vi "example_main.vi"() -> ()   [LabVIEW 2015]
doc: "# #############################################################################\n# ATTENTION\n# #############################################################################\n#\n# This software is for guidance only. It is provided \"as is\".\n# It only aims at providing coding information to the customer in order for\n# them to save time. As a result no warranties, whether express, implied or\n# statutory, including, but not limited to implied warranties of\n# merchantability and fitness for a particular purpose apply to this software.\n# A·P·E Angewandte Physik und Elektronik GmbH shall not be held liable for any\n# direct, indirect or consequential damages with respect to any claims arising\n# from the content of such sourcecode and/or the use made by customers of the\n# coding information contained herein in connection with their products.\n#\n# File Version: 1.0\n#\n# Changelog:\n# 1.0 - Initial Version\n#\n# #############################################################################"
uses:
  <vilib>/Utility/miscctls.llb/LVPointTypeDef.ctl
  cluster/tcp client action.ctl
panel:
  in  "error in":errorcluster
  out "error out":errorcluster
  in  "Send":bool
  out "Answer":string
  in  "Command":string="*IDN?\n"
  in  "Connect":bool
  in  "Host":string="127.0.0.1"
  in  "Port":u16=51019
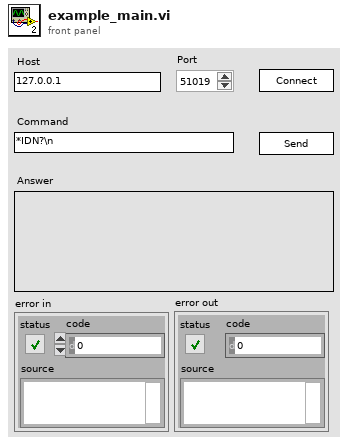
[diagram p1: front panel]
types:
  T1 = typedef "LVPointTypeDef.ctl" = cluster{"Horizontal":i16, "Vertical":i16}
  T2 = typedef "tcp client action.ctl" = enum16{"Connect", "Write", "Query", "Disconnect"}
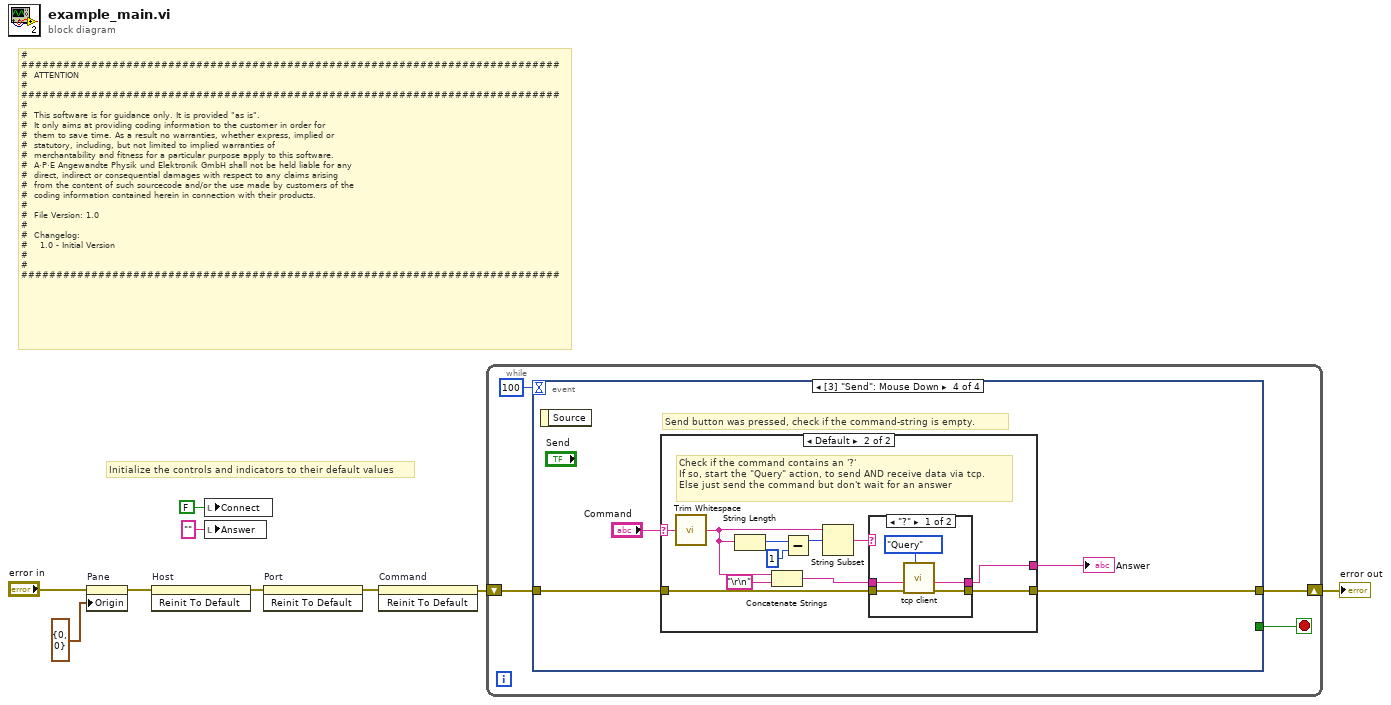
[diagram p0: block diagram]
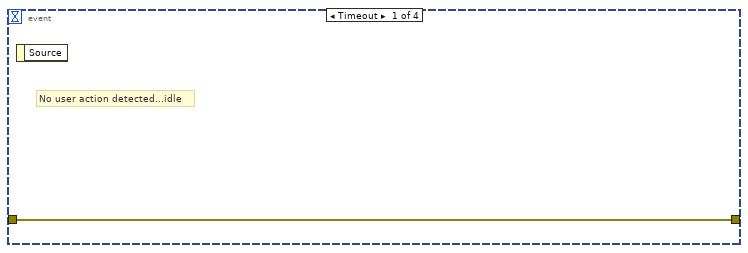
[diagram p2: hidden frame]
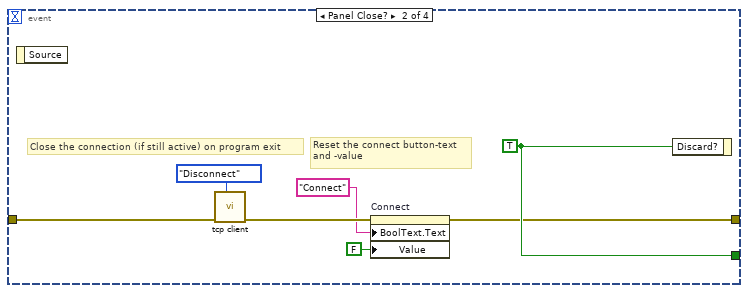
[diagram p3: hidden frame]
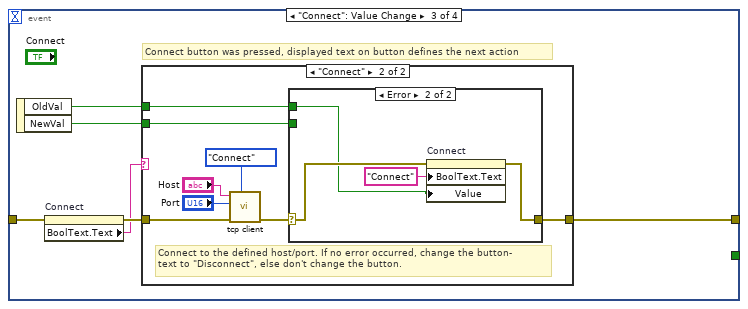
[diagram p4: hidden frame]
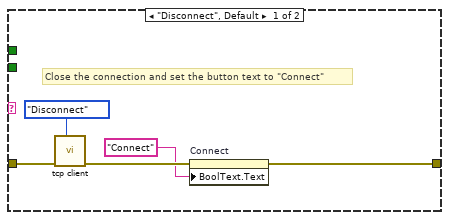
[diagram p5: hidden frame]
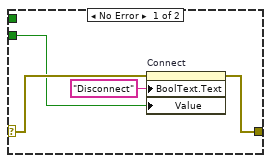
[diagram p6: hidden frame]
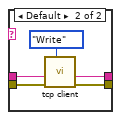
[diagram p8: hidden frame]
diagram:
  # "# #############################################################################\n#  ATTENTION\n# #############################################################################\n#\n#  This software is for guidance only. It is provided \"as is\".\n#  It only aims at providing coding information to the customer in order for\n#  them to save time. As a result no warranties, whether express, implied or\n#  statutory, including, but not limited to implied warranties of\n#  merchantability and fitness for a particular purpose apply to this software.\n#  A·P·E Angewandte Physik und Elektronik GmbH shall not be held liable for any\n#  direct, indirect or consequential damages with respect to any claims arising\n#  from the content of such sourcecode and/or the use made by customers of the\n#  coding information contained herein in connection with their products.\n#\n#  File Version: 1.0\n#\n#  Changelog:\n#    1.0 - Initial Version\n#\n# #############################################################################"
  # "Initialize the controls and indicators to their default values"
  n1 = property on="Pane" class="Pane"(error in="error in", "Origin"=T1 {"Horizontal"=0, "Vertical"=0}) -> (error out=w2:errorcluster)  [unwired: 1 in, 1 out]
  n2 = invoke on="Host" class="Str" method="Reinit To Default"(error in=w2) -> (error out=w5:errorcluster)  [unwired: 2 in, 2 out]
  n3 = local write "Connect"(FALSE ("Connect")) -> ()
  n4 = local write "Answer"("" ("Answer")) -> ()
  n5 = invoke on="Port" class="DigNum (strict)" method="Reinit To Default"(error in=w5) -> (error out=w4:errorcluster)  [unwired: 2 in, 2 out]
  n6 = invoke on="Command" class="Str" method="Reinit To Default"(error in=w4) -> (error out=w3:errorcluster)  [unwired: 2 in, 2 out]
  n7 = while {
    shift-right: [w12] -> w9
    shift-left: w3 -> [w11]
    stop <- w10 stop-if-true
    n8 = event shown="[3] \"Send\": Mouse Down" {
      selector: _ -> [_ _ _ _]
      dyn-events: _ -> [_ _ _ _]
      timeout: 100 -> [_ _ _ _]
      tunnel: w11 -> [w14 w21 w26 w52]
      tunnel: [w14 w17 w27 w49] -> w12
      tunnel: [_ w19 _ _] -> w10
      event Timeout {
        # "No user action detected...idle"
        n9 = event-data() -> ()  [unwired: 1 in, 1 out]
      }
      event Panel Close? {
        w19 = TRUE ("Discard?")
        # "Reset the connect button-text\nand -value"
        # "Close the connection (if still active) on program exit"
        n10 = event-data() -> ()  [unwired: 1 in, 1 out]
        n11 = call "tcp client.vi"("Action"=tcp_client_action."Disconnect", "error in"=w21) -> ("error out"=w18:errorcluster)  [unwired: 8 in, 1 out]
        n12 = property on="Connect" class="Bool (strict)"(error in=w18, "BoolText.Text"="Connect" ("Boolean Text.Text"), "Value"=FALSE ("Connect")) -> (error out=w17:errorcluster)  [unwired: 1 in, 1 out]
        n13 = event-data("Discard?"=w19) -> ()  [unwired: 1 in, 1 out]
      }
      event "Connect": Value Change {
        # "Connect button was pressed, displayed text on button defines the next action"
        n14 = event-data() -> ("OldVal"=w22:bool, "NewVal"=w23:bool)  [unwired: 1 in]
        n15 = property on="Connect" class="Bool (strict)"(error in=w26) -> (error out=w25:errorcluster, "BoolText.Text"=w24:string)  [unwired: 1 in, 1 out]
        n16 = case shown="\"Connect\"" w24 {
          tunnel: [w29 w36] -> w27
          tunnel: w25 -> [w31 w37]
          tunnel: w23 -> [_ w34]
          tunnel: w22 -> [_ w33]
          frame "Disconnect", Default {
            # "Close the connection and set the button text to \"Connect\""
            n17 = call "tcp client.vi"("Action"=tcp_client_action."Disconnect", "error in"=w31) -> ("error out"=w30:errorcluster)  [unwired: 8 in, 1 out]
            n18 = property on="Connect" class="Bool (strict)"(error in=w30, "BoolText.Text"="Connect" ("Boolean Text.Text")) -> (error out=w29:errorcluster)  [unwired: 1 in, 1 out]
          }
          frame "Connect" {
            # "Connect to the defined host/port. If no error occurred, change the button-\ntext to \"Disconnect\", else don't change the button."
            n19 = call "tcp client.vi"("Action"=tcp_client_action."Connect", "error in"=w37, "TCP Port"="Port", "Host"="Host") -> ("error out"=w35:errorcluster)  [unwired: 6 in, 1 out]
            n20 = case shown="Error" w35 {
              selector: w35 -> [w43 w47]
              tunnel: [w44 w48] -> w36
              tunnel: w34 -> [w41 _]
              tunnel: w33 -> [_ w45]
              frame No Error {
                n21 = property on="Connect" class="Bool (strict)"(error in=w43, "BoolText.Text"="Disconnect" ("Boolean Text.Text"), "Value"=w41) -> (error out=w44:errorcluster)  [unwired: 1 in, 1 out]
              }
              frame Error {
                n22 = property on="Connect" class="Bool (strict)"(error in=w47, "BoolText.Text"="Connect" ("Boolean Text.Text"), "Value"=w45) -> (error out=w48:errorcluster)  [unwired: 1 in, 1 out]
              }
            }
          }
        }
      }
      event "Send": Mouse Down {
        # "Send button was pressed, check if the command-string is empty."
        n23 = event-data() -> ()  [unwired: 1 in, 1 out]
        n24 = case shown="Default" "Command" {
          selector: "Command" -> [_ w54]
          tunnel: w52 -> [w53 w60]
          tunnel: [w53 w59] -> w49
          tunnel: [_ w57] -> w50
          frame "" {
            # "Command-string is empty - do nothing"
          }
          frame Default {
            # "Check if the command contains an '?'\nIf so, start the \"Query\" action, to send AND receive data via tcp.\nElse just send the command but don't wait for an answer"
            n25 = call <vilib>:"Trim Whitespace.vi"("string"=w54) -> ("trimmed string"=w58:string)  [unwired: 1 in]
            n26 = String Length(string=w58) -> (length=w63:i32)
            n27 = Concatenate Strings(w58, "\r\n") -> (w56:string)
            n28 = Subtract(x=w63, y=1) -> (x-y=w62:i32)
            n29 = String Subset(string=w58, offset (0)=w62) -> (substring=w61:string)  [unwired: 1 in]
            n30 = case shown="\"?\"" w61 {
              tunnel: [w68 w73] -> w57
              tunnel: [w66 w72] -> w59
              tunnel: w60 -> [w67 w71]
              tunnel: w56 -> [w65 w70]
              frame "?" {
                n31 = call "tcp client.vi"("Action"=tcp_client_action."Query", "error in"=w67, "Command"=w65) -> ("error out"=w66:errorcluster, "Answer"=w68:string)  [unwired: 7 in]
              }
              frame Default {
                n32 = call "tcp client.vi"("Action"=tcp_client_action."Write", "error in"=w71, "Command"=w70) -> ("error out"=w72:errorcluster, "Answer"=w73:string)  [unwired: 7 in]
              }
            }
          }
        }
        "Answer" <- w50
      }
    }
  }
  "error out" <- w9
